vi "Mix Audio.vi"(8 "Array 2":sgl[](array[numeric]), 9 "Array 1":sgl[](array[numeric])) -> (1 "Array out":sgl[](array[numeric]))   [LabVIEW 2015]
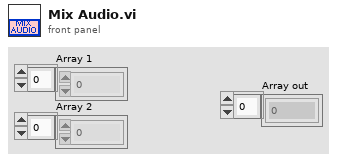
[diagram p1: front panel]
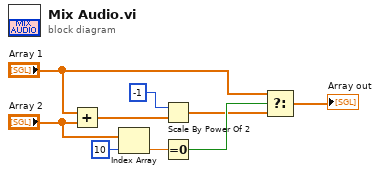
[diagram p0: block diagram]
diagram:
  n1 = Add(x="Array 1", y="Array 2") -> (x+y=w8:sgl[])
  n2 = Index Array(array="Array 2", index=10) -> (element=w5:sgl)
  n3 = Scale By Power Of 2(n=i16 -1, x=w8) -> (x*2^n=w1:sgl[])
  n4 = Equal To 0?(x=w5) -> (x = 0?=w4:bool)
  n5 = Select(t="Array 1", s=w4, f=w1) -> (s? t:f=→"Array out":sgl[])
